vi "Untitled 12.vi"() -> ()   [LabVIEW 2017]
uses:
  a171be36-dab3-4979-9ec1-47a5813348d9.vi
  API-String-Arugments-Support/_Support/Convert API String Arguments to Data(variant).vi
panel:
  out "Cluster":cluster{"2d":dbl[][]}={"2d"=[[3.12, 4.113, 2.3, 5.0, 5.0, 2.3, 4.11, 5.0]]}
  out "error 13":errorcluster
  in  "String 13":string="[3.12,4.113,2.3,5;3.12,5,2.3;3.12,4.11,5]"
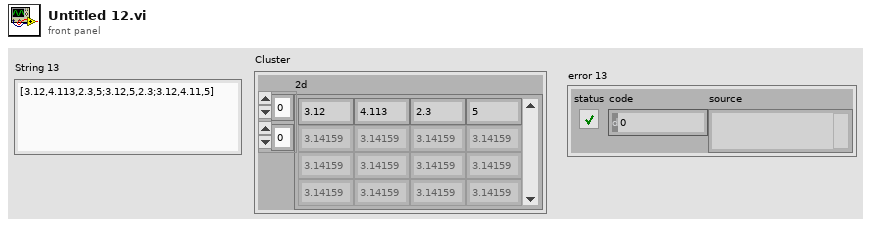
[diagram p1: front panel]
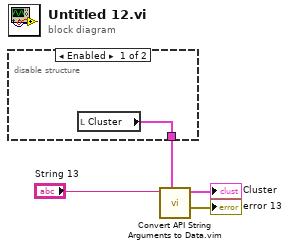
[diagram p0: block diagram]
diagram:
  n1 = disable-structure shown="Enabled" {
    disable-tunnel: [w5 _] -> w2
    frame Enabled {
      n2 = local read "Cluster"() -> (w5:cluster{"2d":dbl[][]})
    }
    frame Disabled {
    }
  }
  n3 = call "Convert API String Arguments to Data.vim"("Type"=w2, "String"="String 13") -> ("error"=→"error 13":errorcluster, "Data"=→"Cluster":cluster{"2d":dbl[][]})  [unwired: 6 in]
